vi "uTransport_uActor_Dequeue.vi"(8 "error in (no error)":errorcluster, 9 "timeout in ms (-1)":i32, 11 "uTransport_uActor in":refnum<class "uTransport_uActor.lvclass">) -> (0 "error out":errorcluster, 2 "Msg":refnum<class "uMsg.lvclass">)   [LabVIEW 2023, in "uFramework.lvlib" / "uTransport_uActor.lvclass"]
doc: "Dequeue an element or return error 550012 on timeout."
uses:
  uTransport_uActor.lvclass
  uMsg/uMsg.lvclass
  uTransport_uActor.lvclass/uTransport_uActor.ctl
  <vilib>/Utility/error.llb/Error Cluster From Error Code.vi
  <vilib>/ErrorRing/Error Ring.xnode
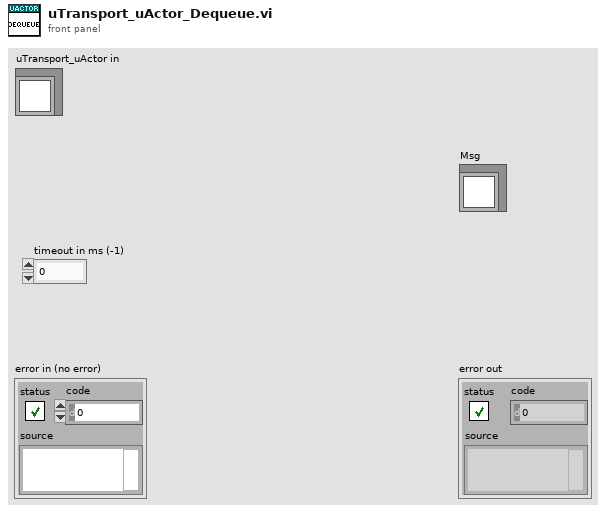
[diagram p1: front panel]
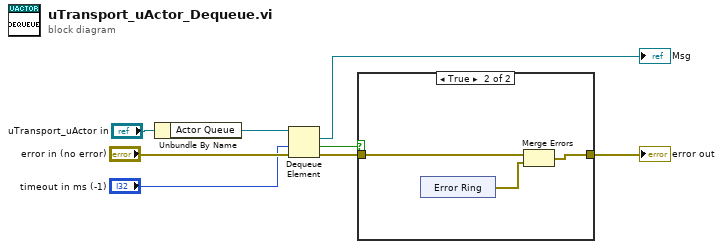
[diagram p0: block diagram]
diagram:
  n1 = Unbundle By Name("uTransport_uActor in") -> ("Actor Queue"=w1:refnum<queue>)
  n2 = Dequeue Element(queue=w1, timeout in ms (-1)="timeout in ms (-1)", error in (no error)="error in (no error)") -> (element=→"Msg":refnum<class "uMsg.lvclass">, timed out?=w4:bool, error out=w2:errorcluster)  [unwired: 1 out]
  n3 = case shown="True" w4 {
    tunnel: [w9 w11] -> w3
    tunnel: w2 -> [w9 w12]
    frame False {
    }
    frame True {
      n4 = xnode "Error Ring"() -> ("error out"=w10:errorcluster)
      n5 = Merge Errors(w12, w10) -> (w11:errorcluster)
    }
  }
  "error out" <- w3
